vi "Export_Get Export File Setting.vi"(11 "Device Export Setup":T2) -> (3 "Export File Setting":T1)   [LabVIEW 2015, in "ConfigHelper.lvlib"]
uses:
  ConfigHelper.lvlib
  Control_Export Setup.ctl
  Control_Export File Setup.ctl
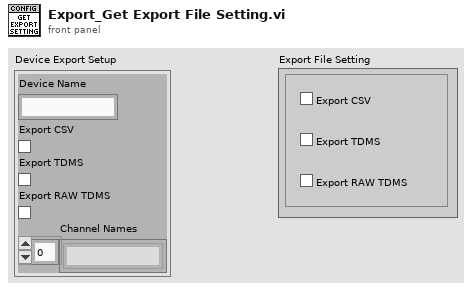
[diagram p1: front panel]
types:
  T1 = typedef "ConfigHelper.lvlib/Control_Export File Setup.ctl" = cluster{"CSV":bool, "TDMS":bool, "RAW TDMS":bool}
  T2 = typedef "ConfigHelper.lvlib/Control_Export Setup.ctl" = cluster{"Device Name":string, "Export CSV":bool, "Export TDMS":bool, "Export RAW TDMS":bool, "Channel Names":string[]}
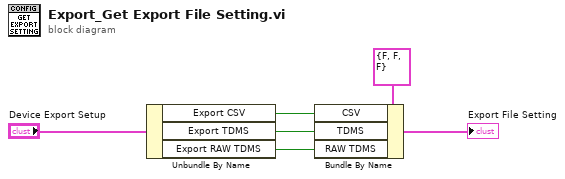
[diagram p0: block diagram]
diagram:
  n1 = Unbundle By Name("Device Export Setup") -> ("Export CSV"=w4:bool, "Export TDMS"=w3:bool, "Export RAW TDMS"=w2:bool)
  n2 = Bundle By Name(cluster=T1 {"CSV"=FALSE, "TDMS"=FALSE, "RAW TDMS"=FALSE} ("Export File Setup"), "CSV"=w4, "TDMS"=w3, "RAW TDMS"=w2) -> (→"Export File Setting":T1)
